vi "Channel by Index.vi"(8 "error in (no error)":errorcluster, 10 "Index":i32, 11 "StringGroup in":refnum<class "StringGroup.lvclass">) -> (0 "error out":errorcluster, 2 "StringChannel":refnum<class "StringChannel.lvclass">, 3 "StringGroup out":refnum<class "StringGroup.lvclass">)   [LabVIEW 2020, in "Vecto.lvlib" / "StringGroup.lvclass"]
uses:
  StringGroup.lvclass
  StringChannel/StringChannel.lvclass
  StringGroup.lvclass/StringGroup.ctl
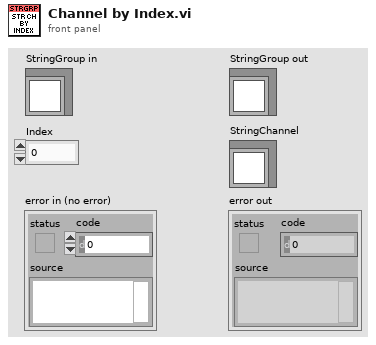
[diagram p1: front panel]
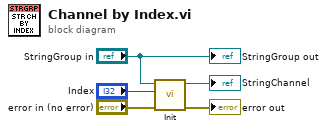
[diagram p0: block diagram]
diagram:
  n1 = call "Init.vi"("error in (no error)"="error in (no error)", "Index"="Index", "Group"="StringGroup in") -> ("error out"=→"error out":errorcluster, "StringChannel out"=→"StringChannel":refnum<class "StringChannel.lvclass">)  [unwired: 7 in]
  "StringGroup out" <- "StringGroup in"
